vi "CloseRelay.vi"(8 "error in (no error)":errorcluster, 11 "Relay Identifier":i32=349111800) -> (0 "error out":errorcluster)   [LabVIEW 2022 SP3, in "usb_relay_device.lvlib"]
doc: "void EXPORT_API usb_relay_device_close(int hHandle);"
uses:
  usb_relay_device.lvlib
  usb_relay_device.dll
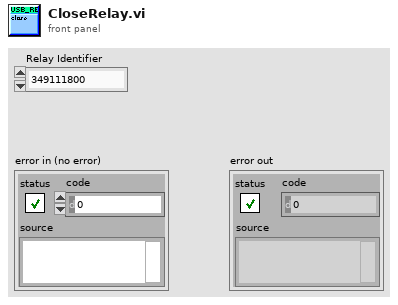
[diagram p1: front panel]
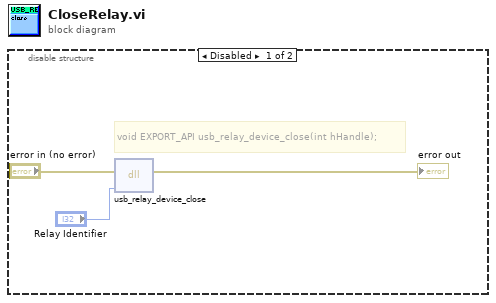
[diagram p0: block diagram]
diagram:
  n1 = disable-structure shown="Disabled" {
    frame Disabled {
      # "void EXPORT_API usb_relay_device_close(int hHandle);"
      n2 = dll-call lib="D:/LabVIEWSuite_64_OS/ScanningControl/Switch Modules/RiversideUSBRealy/usb_relay_device.*" fn="usb_relay_device_close"(error in="error in (no error)", "hHandle"="Relay Identifier") -> (error out=→"error out":errorcluster)  [unwired: 4 in, 1 out]
    }
    frame Enabled {
    }
  }
